vi "NHMFL TL Front Panel.vi"() -> ()   [LabVIEW 2020]
panel:
  out "Temp Display":enum32{"Helium 3", "VTI"}(tab)
  out "SORB":dbl
  out "1K POT":dbl
  out "3HE POT":dbl
  out "PROBE":dbl
  out "SAMPLE":dbl
  out "VTI":dbl
  in  "Load Probe Step Number":u8
  in  "Initialize":bool
  out "Array":dbl[][](array[numeric])
  in  "Menu Button":bool
  out "Tab Control":T1(tab)=enum."Menu"
  in  "Configure Instruments":bool
  in  "Choose Insert":enum32{"Helium 3", "VTI"}(radio)
  in  "Choose System":T2(radio)
  in  "Ring":u16(ring)=1 items=["Choose Function"=1, "He3 Condense"=3, "Change Setpoint"=8, "Temperature Ramp"=4]
  in  "stop":bool
  out "Load Probe Prompt":string
  in  "Load Probe: Next Step":bool
  out "Load Probe: Status":string
  in  "Quick Condense":bool
  in  "Condense Followup":u16(ring) items=["What Next?", "Hold @ 45K", "Run to Base", "Begin Ramp"]
  in  "Condense Continue Button":bool
  out "Position":string
  in  "Prior":bool
  in  "Next":bool
  in  "Soak Time":dbl format="%<%H:%M:%S>t"
  in  "Ramp Time":dbl format="%<%H:%M:%S>t"
  in  "Target Temp":dbl min=0.0 max=45.0 step=0.0001
  in  "Run Button":bool
  in  "Reset Button":bool
  out "Temp Array":dbl[](array[numeric])
  out "Time Array":dbl[][](array[numeric]) format="%<%H:%M:%S>t"
  in  "Proportional":sgl=1000.0 min=0 max=1000 step=0.1
  in  "Integral":sgl min=0 max=1000 step=0.1
  in  "Derivative":sgl min=0 max=1000 step=1
  out "Derivative Default":sgl
  out "Integral Default":sgl
  out "Proportional Default":sgl
  in  "Submit PID":bool
  in  "Probe Setpoint":dbl min=0.0 max=1.483 step=1e-05
  in  "Sorb Setpoint":dbl min=0.0 max=45.0 step=1e-05
  in  "Submit Setpoint":bool
  # "He3 Condensation:\n   Choose Full (1 hour) or Quick (30 min)\nCondense, then select a routine to start \nonce the helium has condensed."
  # "Condense,"
  # "then"
  # "Enter Target Sample Temperatures"
  # "Default"
  # "Change setpoint to what value?"
  # "≈"
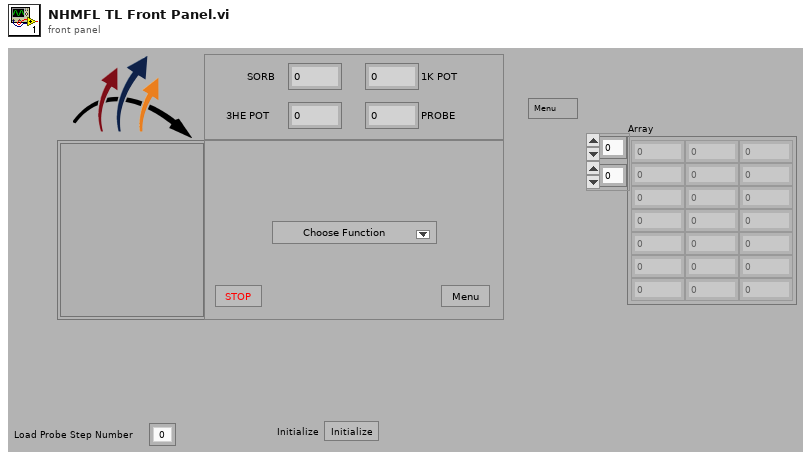
[diagram p1: front panel]
types:
  T1 = enum32{"Identify System", "Menu", "Load Probe", "He3 Condense", "Temperature Ramp", "Ramp Aray", "PID Control", "Configure Instruments", "Change Setpoint"}
  T2 = enum32{"TL-SC  (System A)", "SIV-32 (System B)", "TL-50  (System C)", "TL-32  (System D)"}
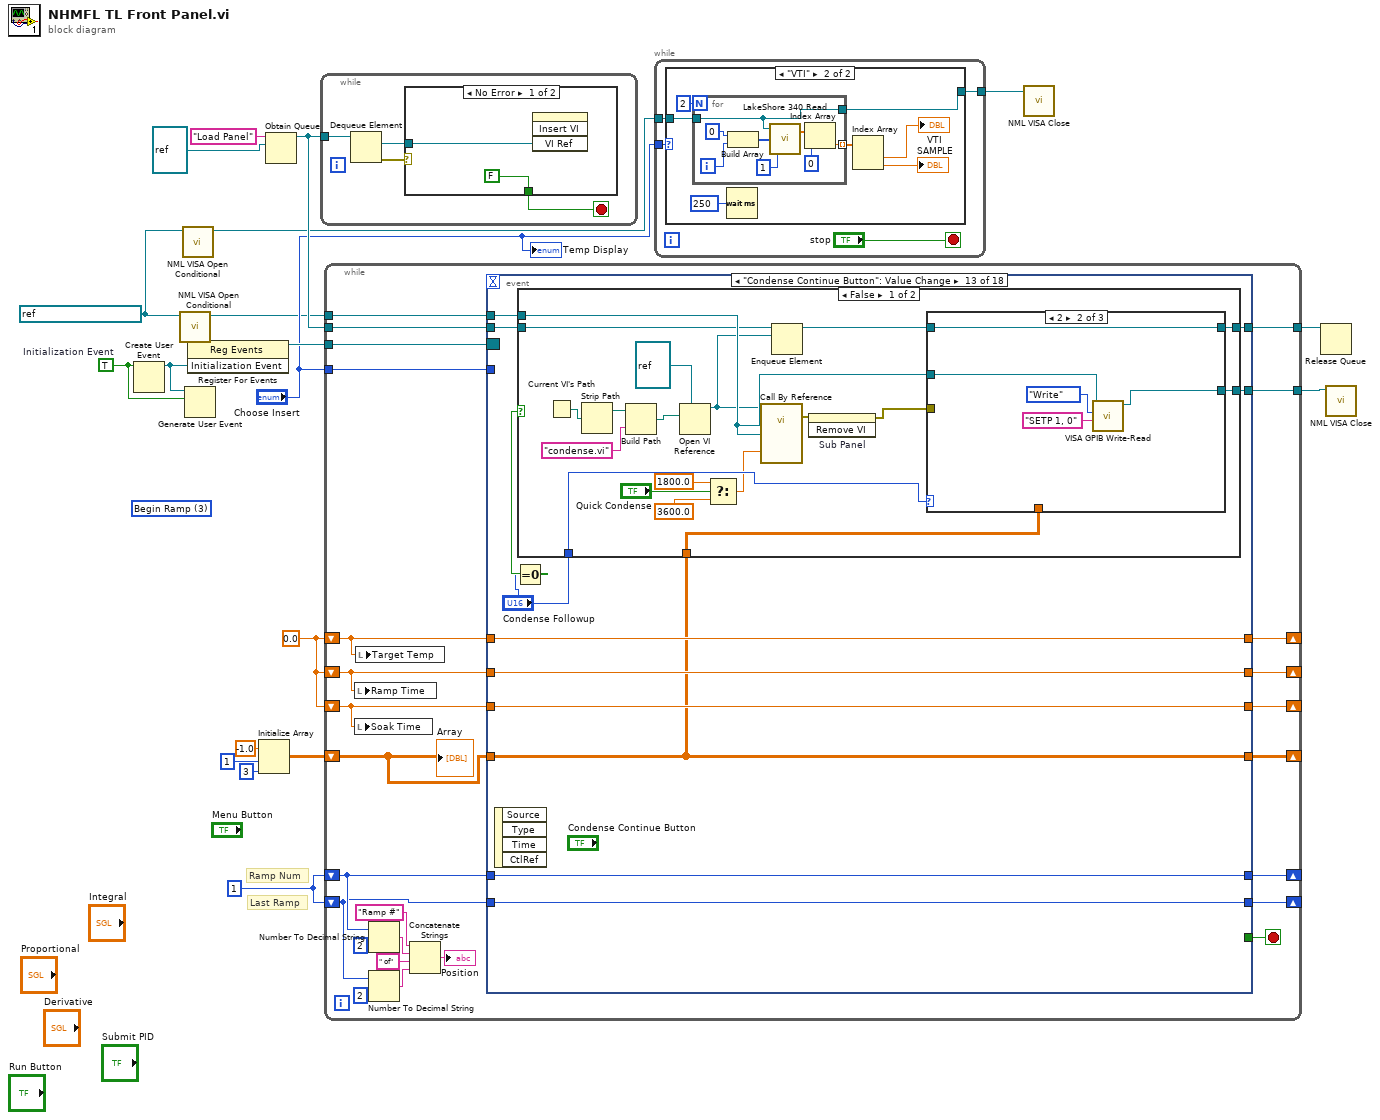
[diagram p0: block diagram]
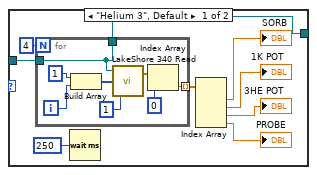
[diagram p2: hidden frame]
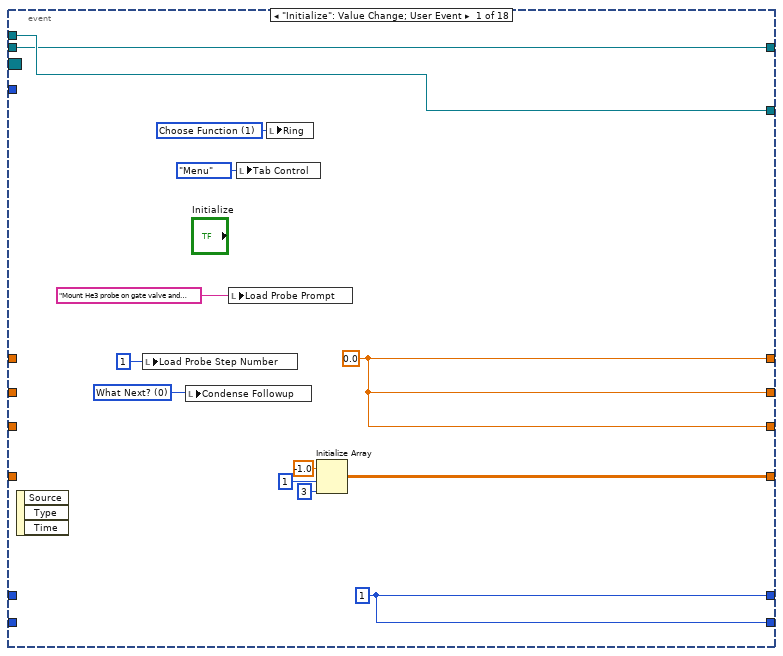
[diagram p3: hidden frame]
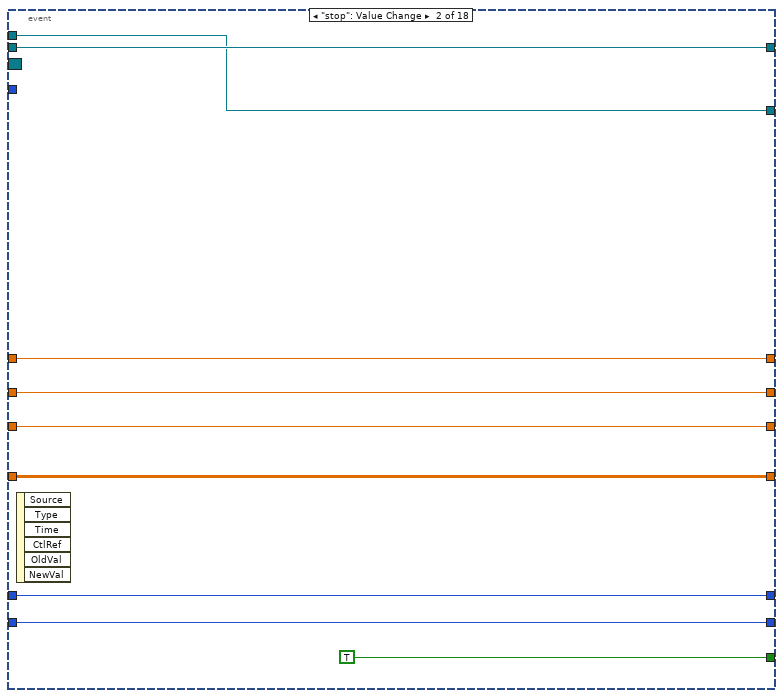
[diagram p4: hidden frame]
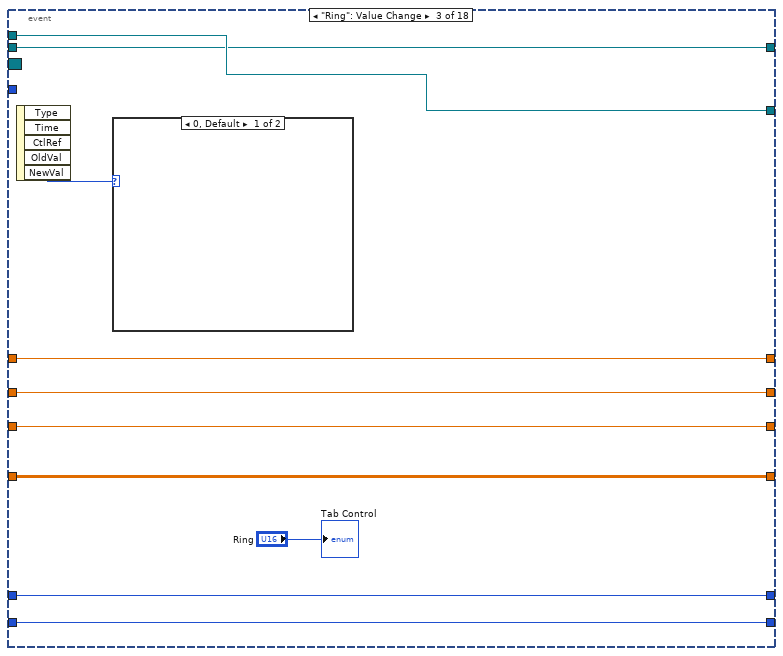
[diagram p5: hidden frame]
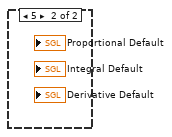
[diagram p6: hidden frame]
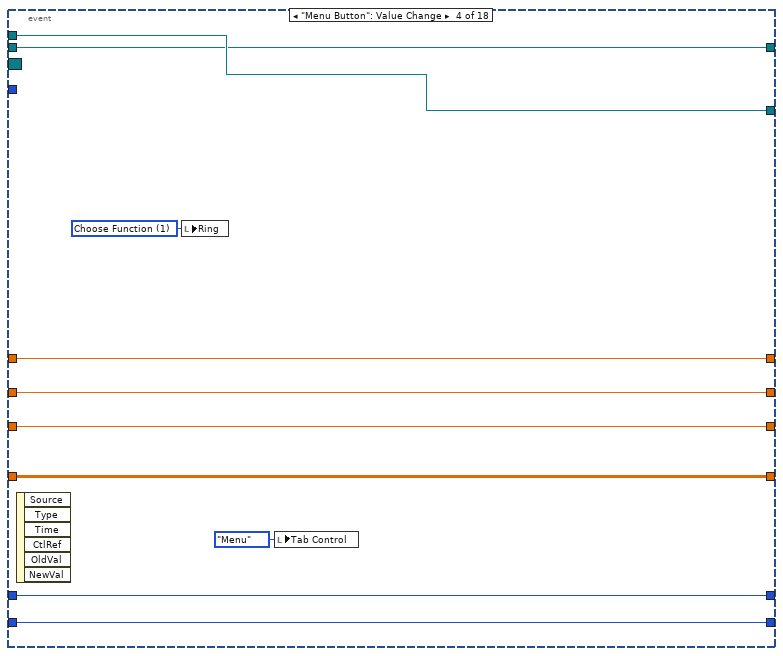
[diagram p7: hidden frame]
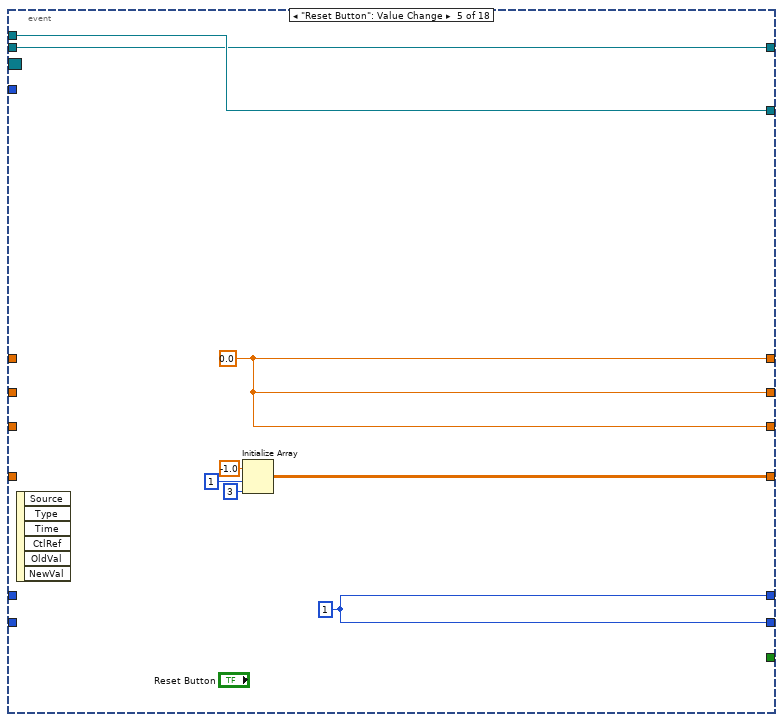
[diagram p8: hidden frame]
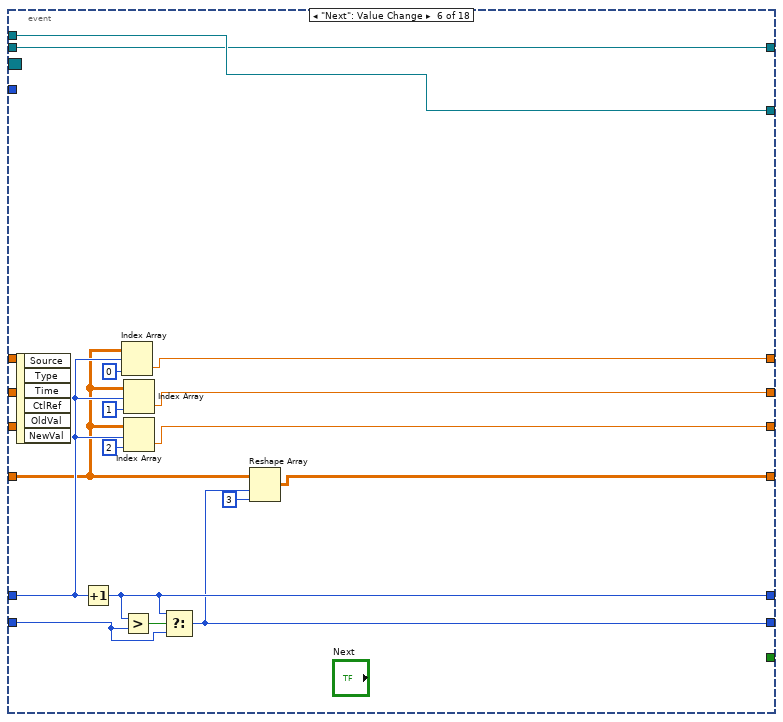
[diagram p9: hidden frame]
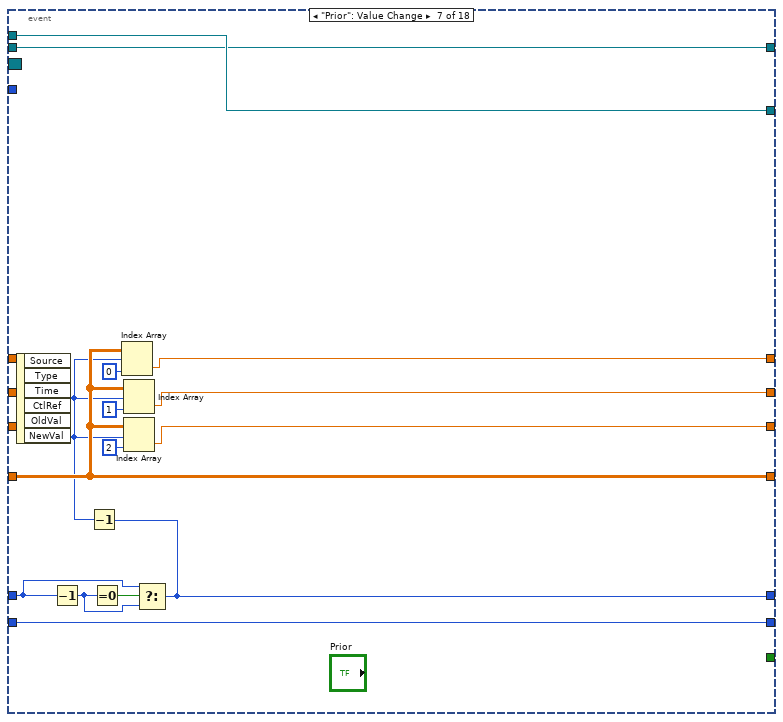
[diagram p10: hidden frame]
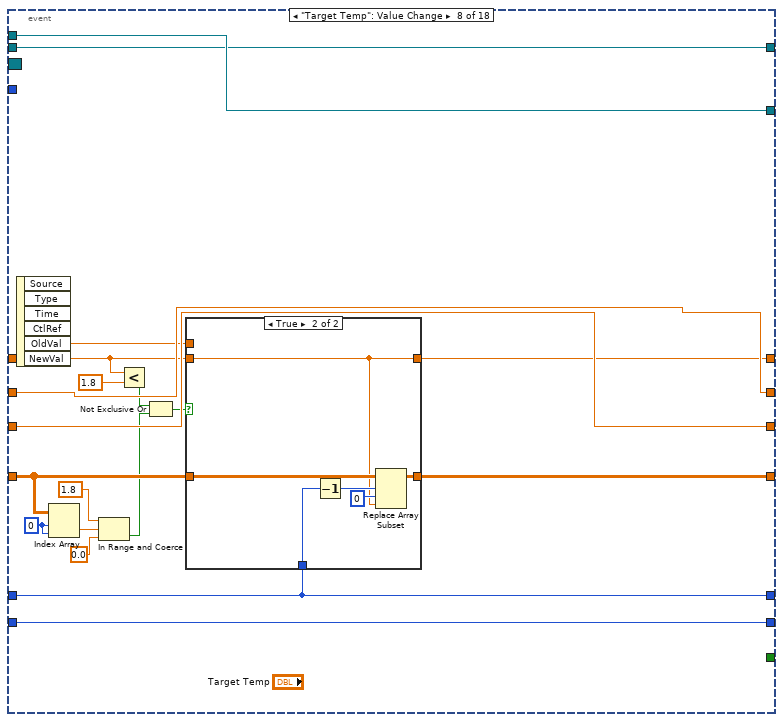
[diagram p11: hidden frame]
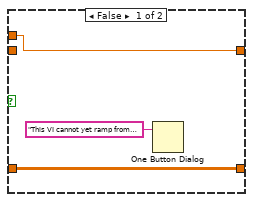
[diagram p12: hidden frame]
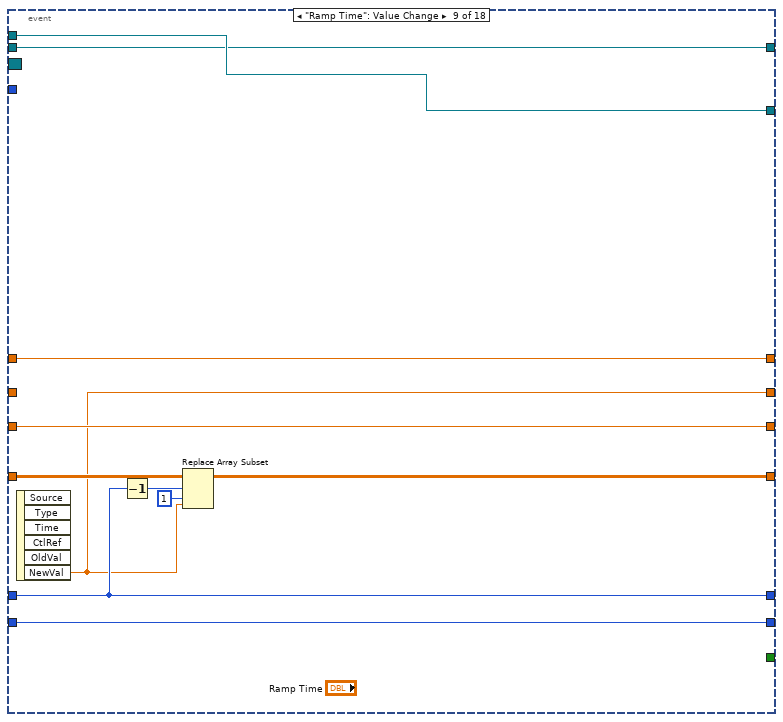
[diagram p13: hidden frame]
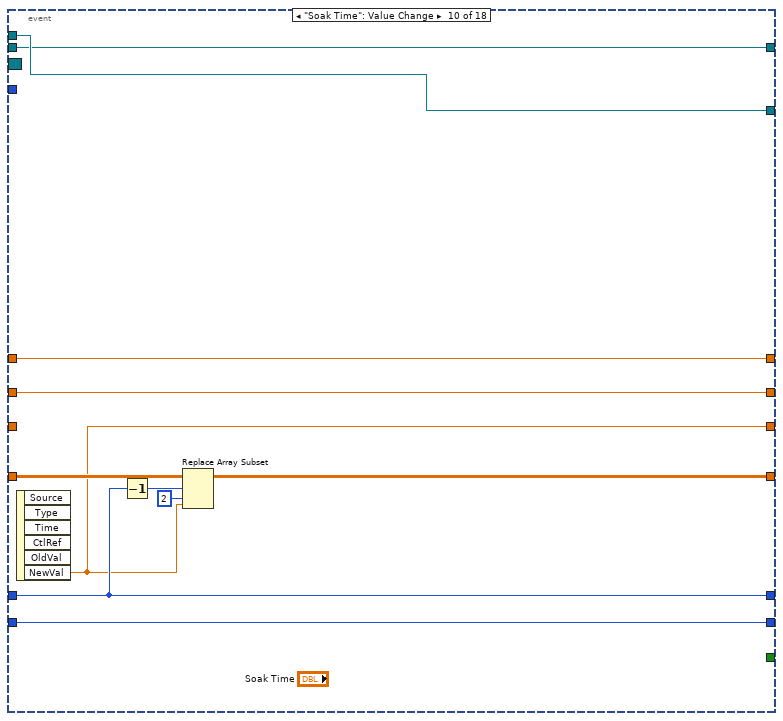
[diagram p14: hidden frame]
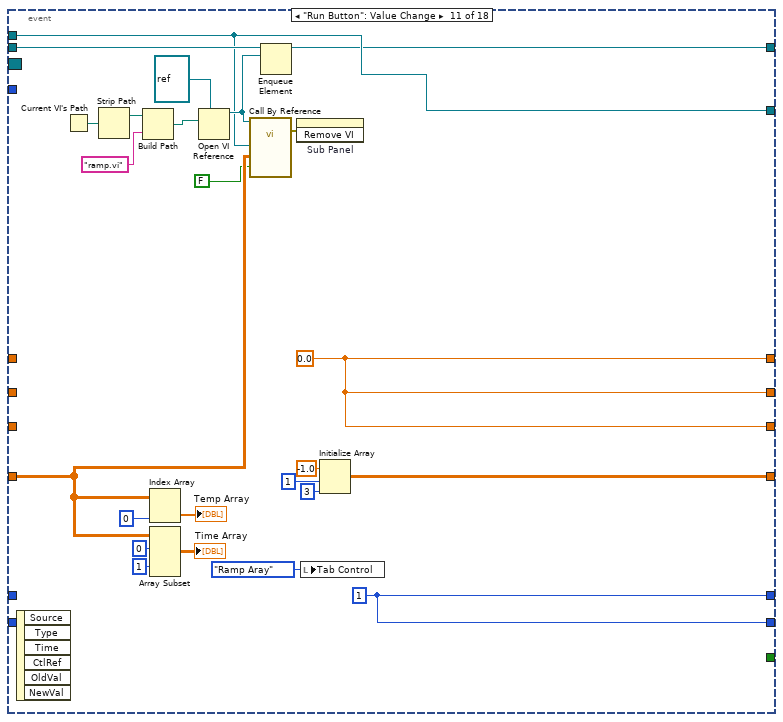
[diagram p15: hidden frame]
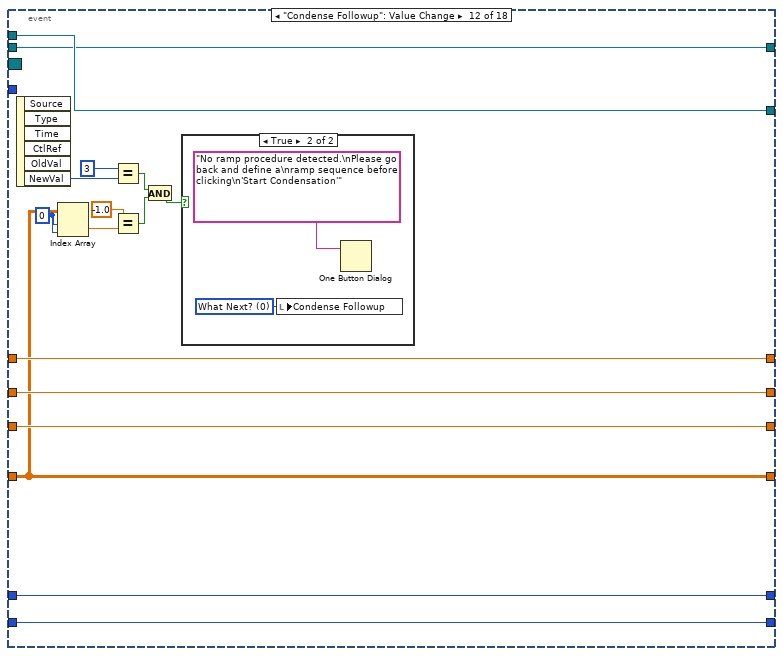
[diagram p16: hidden frame]
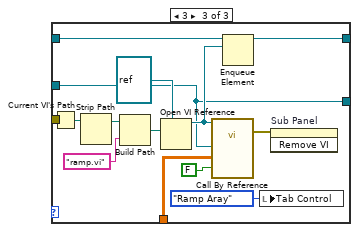
[diagram p19: hidden frame]
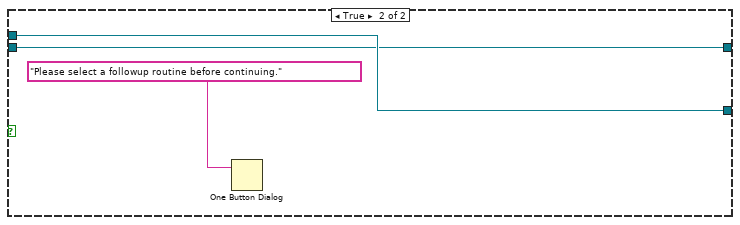
[diagram p20: hidden frame]
diagram:
  (unwired) u16 3 items=["What Next?", "Hold @ 40K", "Run to Base", "Begin Ramp"] ("Condense Followup")
  w7 = TRUE  # Initialization Event
  w6 = refnum<visa-resource-name> "GPIB0::12::INSTR" ("Instrument Address")
  w11 = u8 1
  w16 = 0.0 ("Target Temp")
  # "Last Ramp"
  # "Ramp Num"
  n1 = Create User Event(user event datatype=w7) -> (user event=w8:refnum<user-event>)  [unwired: 1 in, 1 out]
  n2 = call "NML VISA Open Conditional.vi"("VISA resource name"=w6) -> ("dup VISA Session"=w3:refnum<visa-resource-name>)  [unwired: 8 in, 2 out]
  n3 = call "NML VISA Open Conditional.vi"("VISA resource name"=w6) -> ("dup VISA Session"=w4:refnum<visa-resource-name>)  [unwired: 8 in, 2 out]
  n4 = Generate User Event(user event=w8, event data cluster=w7) -> ()  [unwired: 2 in, 2 out]
  n5 = register-events(w8) -> (reference out=w9:refnum<event-registration>)  [unwired: 2 in, 1 out]
  n6 = Initialize Array(-1.0 ("element"), 1 ("dimension size"), 3 ("dimension size")) -> (w12:dbl[][])
  n7 = Obtain Queue(name (unnamed)="Load Panel", element data type=refnum<vi> refnum ("vi reference")) -> (queue out=w17:refnum<queue>)  [unwired: 3 in, 2 out]
  n8 = while {
    tunnel: w17 -> [w23]
    stop <- w20 stop-if-true
    n9 = Dequeue Element(queue=w23) -> (element=w21:refnum<vi>, error out=w22:errorcluster)  [unwired: 2 in, 2 out]
    n10 = case shown="No Error" w22 {
      tunnel: w21 -> [w24 _]
      tunnel: [FALSE TRUE] -> w20
      frame No Error {
        n11 = invoke on="Sub Panel" class="SubPnl" method="Insert VI"("VI Ref"=w24) -> ()  [unwired: 3 in, 4 out]
      }
      frame Error {
      }
    }
  }
  n12 = while {
    tunnel: w17 -> [w33]
    shift-right: [w49] -> _
    shift-left: w12 -> [w31]
    shift-right: [w47] -> _
    shift-left: w16 -> [w50]
    shift-right: [w48] -> _
    shift-left: w16 -> [w51]
    shift-right: [w46] -> _
    shift-left: w16 -> [w52]
    shift-right: [w45] -> _
    shift-left: w11 -> [w36]
    shift-right: [w44] -> _
    shift-left: w11 -> [w35]
    tunnel: [w32] -> w10
    tunnel: w3 -> [w30]
    tunnel: w9 -> [w29]
    tunnel: "Choose Insert" -> [w28]
    tunnel: [w27] -> w1
    stop <- w34 stop-if-true
    n13 = local write "Ramp Time"(w51) -> ()
    n14 = local write "Soak Time"(w50) -> ()
    n15 = local write "Target Temp"(w52) -> ()
    n16 = Number To Decimal String(number=w36, width (-)=i16 2) -> (decimal integer string=w39:string)
    n17 = Number To Decimal String(number=w35, width (-)=i16 2) -> (decimal integer string=w37:string)
    n18 = Concatenate Strings("Ramp #", w39, " of", w37) -> (→"Position":string)
    n19 = event shown="[12] \"Condense Continue Button\": Value Change" {
      selector: w29 -> [_ _ _ _ _ _ _ _ _ _ _ _ _ _ _ _ _ _]
      dyn-events: _ -> [_ _ _ _ _ _ _ _ _ _ _ _ _ _ _ _ _ _]
      timeout: _ -> [_ _ _ _ _ _ _ _ _ _ _ _ _ _ _ _ _ _]
      tunnel: w51 -> [_ w70 w83 w93 _ _ _ w152 _ w176 _ w222 w233 w293 w325 w334 w344 w360]
      tunnel: w50 -> [_ w69 w82 w92 _ _ _ w151 w172 _ _ w221 w234 w292 w324 w333 w343 w359]
      tunnel: w52 -> [_ w71 w84 w94 _ _ _ _ w165 w177 _ w223 w232 w294 w326 w335 w345 w361]
      tunnel: w31 -> [_ w68 w81 w91 _ w105 w126 w147 w171 w183 w195 w216 w230 w291 w323 w332 w342 w358]
      tunnel: [w61 w68 w81 w91 w99 w109 w126 w150 w170 w182 w188 w216 w230 w291 w323 w332 w342 w358] -> w49
      tunnel: [w65 w70 w83 w93 w98 w107 w129 w152 w164 w176 w189 w222 w233 w293 w325 w334 w344 w360] -> w48
      tunnel: [w65 w69 w82 w92 w98 w115 w130 w151 w172 w175 w189 w221 w234 w292 w324 w333 w343 w359] -> w47
      tunnel: [w65 w71 w84 w94 w98 w106 w128 w140 w165 w177 w189 w223 w232 w294 w326 w335 w345 w361] -> w46
      tunnel: w35 -> [_ w66 w79 w89 _ w113 w127 w148 w166 w178 _ w219 w236 w289 w321 w330 w340 w356]
      tunnel: w36 -> [_ w67 w80 w90 _ w112 w124 w149 w167 w179 _ w220 w237 w290 w322 w331 w341 w357]
      tunnel: [w60 w67 w80 w90 w97 w111 w122 w149 w167 w179 w187 w220 w237 w290 w322 w331 w341 w357] -> w45
      tunnel: [w60 w66 w79 w89 w97 w108 w127 w148 w166 w178 w187 w219 w236 w289 w321 w330 w340 w356] -> w44
      tunnel: [_ TRUE _ _ _ _ _ _ _ _ _ _ _ _ _ _ _ _] -> w34
      tunnel: w33 -> [w53 w73 w75 w85 w95 w103 w119 w134 w162 w173 w196 w208 w235 w280 w312 w328 w338 w348]
      tunnel: [w53 w73 w75 w85 w95 w103 w119 w134 w162 w173 w184 w208 w226 w280 w312 w328 w338 w348] -> w32
      tunnel: w30 -> [w54 w72 w76 w86 w96 w104 w120 w135 w163 w174 w185 w209 w231 w281 w313 w329 w339 w351]
      tunnel: w28 -> [_ _ _ _ _ _ _ _ _ _ _ _ _ _ w318 _ _ _]
      tunnel: [w54 w72 w76 w86 w96 w104 w120 w135 w163 w174 w185 w209 w227 w281 w313 w329 w339 w350] -> w27
      event "Initialize": Value Change; User Event {
        w55 = u16 1 items=["Choose Function"=1, "He3 Condense"=3, "Change Setpoint"=8, "Temperature Ramp"=4] ("Ring")
        w57 = u16 0 items=["What Next?", "Hold @ 45K", "Run to Base", "Begin Ramp"] ("Condense followup")
        w60 = u8 1
        w65 = 0.0 ("Target Temp")
        n20 = event-data() -> ()  [unwired: 1 in, 3 out]
        n21 = local write "Load Probe Step Number"(u8 1 ("Load Probe Step Number")) -> ()
        n22 = local write "Condense Followup"(w57) -> ()
        n23 = local write "Load Probe Prompt"("Mount He3 probe on gate valve and tighten KF-50 clamp." ("Load Probe Prompt")) -> ()
        n24 = local write "Tab Control"(T1."Menu" ("Tab Control")) -> ()
        n25 = local write "Ring"(w55) -> ()
        n26 = Initialize Array(-1.0 ("element"), 1 ("dimension size"), 3 ("dimension size")) -> (w61:dbl[][])
      }
      event "stop": Value Change {
        n27 = event-data() -> ()  [unwired: 1 in, 6 out]
      }
      event "Ring": Value Change {
        n28 = event-data() -> ("NewVal"=w77:u16)  [unwired: 1 in, 4 out]
        n29 = case shown="0, Default" w77 {
          frame 0, Default {
          }
          frame 5 {
          }
        }
        "Tab Control" <- "Ring"
      }
      event "Menu Button": Value Change {
        w87 = u16 1 items=["Choose Function"=1, "He3 Condense"=3, "Change Setpoint"=8, "Temperature Ramp"=4] ("Ring")
        n30 = event-data() -> ()  [unwired: 1 in, 6 out]
        n31 = local write "Ring"(w87) -> ()
        n32 = local write "Tab Control"(T1."Menu" ("Tab Control")) -> ()
      }
      event "Reset Button": Value Change {
        w97 = u8 1
        w98 = 0.0 ("Target Temp")
        n33 = event-data() -> ()  [unwired: 1 in, 6 out]
        n34 = Initialize Array(-1.0 ("element"), 1 ("dimension size"), 3 ("dimension size")) -> (w99:dbl[][])
      }
      event "Next": Value Change {
        n35 = event-data() -> ()  [unwired: 1 in, 6 out]
        n36 = Increment(x=w112) -> (x+1=w111:u8)
        n37 = Index Array(array=w105, index (row)=w112, index (col)=0 ("disabled index (col)")) -> (element=w106:dbl)
        n38 = Greater?(x=w111, y=w113) -> (0:w114:bool)
        n39 = Index Array(array=w105, index (row)=w112, index (col)=1 ("disabled index (col)")) -> (element=w107:dbl)
        n40 = Index Array(array=w105, index (row)=w112, index (col)=2 ("disabled index (col)")) -> (element=w115:dbl)
        n41 = Select(t=w111, s=w114, f=w113) -> (s? t:f=w108:u8)
        n42 = Reshape Array(w105, w108, 3 ("dimension size")) -> (w109:dbl[][])
      }
      event "Prior": Value Change {
        n43 = event-data() -> ()  [unwired: 1 in, 6 out]
        n44 = Decrement(x=w124) -> (x-1=w123:u8)
        n45 = Equal To 0?(x=w123) -> (x = 0?=w125:bool)
        n46 = Select(t=w124, s=w125, f=w123) -> (s? t:f=w122:u8)
        n47 = Decrement(x=w122) -> (x-1=w121:u8)
        n48 = Index Array(array=w126, index (row)=w121, index (col)=0 ("disabled index (col)")) -> (element=w128:dbl)
        n49 = Index Array(array=w126, index (row)=w121, index (col)=1 ("disabled index (col)")) -> (element=w129:dbl)
        n50 = Index Array(array=w126, index (row)=w121, index (col)=2 ("disabled index (col)")) -> (element=w130:dbl)
      }
      event "Target Temp": Value Change {
        w146 = 0 ("index (row)")
        n51 = event-data() -> ("OldVal"=w141:dbl, "NewVal"=w143:dbl)  [unwired: 1 in, 4 out]
        n52 = Index Array(array=w147, index (row)=w146, index (col)=w146) -> (element=w139:dbl)
        n53 = In Range and Coerce(upper limit=1.8 ("y"), x=w139, lower limit=0.0) -> (In Range?=w136:bool)  [unwired: 1 out]
        n54 = Less?(x=w143, y=1.8) -> (x < y?=w144:bool)
        n55 = Not Exclusive Or(1:w136, 2:w144) -> (0:w142:bool)
        n56 = case shown="True" w142 {
          tunnel: [w154 w161] -> w150
          tunnel: w149 -> [_ w160]
          tunnel: w147 -> [w154 w159]
          tunnel: w143 -> [_ w156]
          tunnel: w141 -> [w155 _]
          tunnel: [w155 w156] -> w140
          frame False {
            n57 = One Button Dialog(message="This VI cannot yet ramp from low-temperature (Probe < 1.8K) to high temperature modes.\n\nPlease use two seperate ramp routines.") -> ()  [unwired: 1 in, 1 out]
          }
          frame True {
            n58 = Decrement(x=w160) -> (x-1=w157:u8)
            n59 = Replace Array Subset(array=w159, new element=w156, index (row)=w157, index (col)=0 ("disabled index (col)")) -> (w161:dbl[][])
          }
        }
      }
      event "Ramp Time": Value Change {
        n60 = event-data() -> ("NewVal"=w164:dbl)  [unwired: 1 in, 5 out]
        n61 = Decrement(x=w167) -> (x-1=w168:u8)
        n62 = Replace Array Subset(array=w171, new element=w164, index (row)=w168, index (col)=1 ("disabled index (col)")) -> (w170:dbl[][])
      }
      event "Soak Time": Value Change {
        n63 = event-data() -> ("NewVal"=w175:dbl)  [unwired: 1 in, 5 out]
        n64 = Decrement(x=w179) -> (x-1=w180:u8)
        n65 = Replace Array Subset(array=w183, new element=w175, index (row)=w180, index (col)=2 ("disabled index (col)")) -> (w182:dbl[][])
      }
      event "Run Button": Value Change {
        w187 = u8 1
        w189 = 0.0 ("Target Temp")
        n66 = event-data() -> ()  [unwired: 1 in, 6 out]
        n67 = Current VI's Path() -> (path=w197:path)
        n68 = Strip Path(path=w197) -> (stripped path=w201:path)  [unwired: 1 out]
        n69 = Build Path(base path=w201, name or relative path="ramp.vi") -> (appended path=w200:path)
        n70 = Index Array(array=w195, index (col)=0 ("index (row)")) -> (element=→"Temp Array":dbl[])  [unwired: 1 in]
        n71 = Array Subset(array=w195, index (row)=0, index (col)=1 ("index")) -> (→"Time Array":dbl[][])  [unwired: 2 in]
        n72 = Open VI Reference(type specifier VI Refnum (for type only)=refnum<vi> refnum, vi path=w200) -> (vi reference=w199:refnum<vi>)  [unwired: 4 in, 1 out]
        n73 = call-by-ref "?"(reference=w199, "Log Scale?"=FALSE, "Array"=w195, "Instrument Address"=w185) -> (error out=w194:errorcluster)  [unwired: 1 in, 1 out]
        n74 = Enqueue Element(queue=w196, element=w199) -> (queue out=w184:refnum<queue>)  [unwired: 2 in, 2 out]
        n75 = invoke on="Sub Panel" class="SubPnl" method="Remove VI"(error in=w194) -> ()  [unwired: 2 in, 3 out]
        n76 = local write "Tab Control"(T1."Ramp Aray" ("Tab Control")) -> ()
        n77 = Initialize Array(-1.0 ("element"), 1 ("dimension size"), 3 ("dimension size")) -> (w188:dbl[][])
      }
      event "Condense Followup": Value Change {
        w215 = 0 ("index (row)")
        n78 = event-data() -> ("NewVal"=w218:u16)  [unwired: 1 in, 5 out]
        n79 = Index Array(array=w216, index (row)=w215, index (col)=w215) -> (element=w214:dbl)
        n80 = Equal?(x=u16 3, y=w218) -> (x = y?=w211:bool)
        n81 = Equal?(x=-1.0, y=w214) -> (x = y?=w212:bool)
        n82 = And(x=w211, y=w212) -> (x .and. y?=w210:bool)
        n83 = case shown="True" w210 {
          frame False {
          }
          frame True {
            w224 = u16 0 items=["What Next?", "Hold @ 40K", "Run to Base", "Begin Ramp"] ("Condense Followup")
            n84 = local write "Condense Followup"(w224) -> ()
            n85 = One Button Dialog(message="No ramp procedure detected.\nPlease go back and define a\nramp sequence before clicking\n'Start Condensation'") -> ()  [unwired: 1 in, 1 out]
          }
        }
      }
      event "Condense Continue Button": Value Change {
        n86 = event-data() -> ()  [unwired: 1 in, 4 out]
        n87 = Equal To 0?(x="Condense Followup") -> (x = 0?=w229:bool)
        n88 = case shown="False" w229 {
          tunnel: w235 -> [w240 w277]
          tunnel: w231 -> [w256 w278]
          tunnel: w230 -> [w255 _]
          tunnel: "Condense Followup" -> [w254 _]
          tunnel: [w253 w278] -> w227
          tunnel: [w238 w277] -> w226
          frame False {
            n89 = Current VI's Path() -> (path=w252:path)
            n90 = Strip Path(path=w252) -> (stripped path=w244:path)  [unwired: 1 out]
            n91 = Build Path(base path=w244, name or relative path="condense.vi") -> (appended path=w245:path)
            n92 = Open VI Reference(type specifier VI Refnum (for type only)=refnum<vi> refnum, vi path=w245) -> (vi reference=w250:refnum<vi>)  [unwired: 4 in, 1 out]
            n93 = Select(t=1800.0, s="Quick Condense", f=3600.0 ("t")) -> (s? t:f=w242:dbl)
            n94 = call-by-ref "?"(reference=w250, "Time"=w242, "GPIB Address"=w256) -> (error out=w246:errorcluster)  [unwired: 2 in, 1 out]
            n95 = Enqueue Element(queue=w240, element=w250) -> (queue out=w239:refnum<queue>)  [unwired: 2 in, 2 out]
            n96 = invoke on="Sub Panel" class="SubPnl" method="Remove VI"(error in=w246) -> (error out=w241:errorcluster)  [unwired: 2 in, 2 out]
            n97 = case shown="2" w254 {
              tunnel: w256 -> [w258 w262 w265]
              tunnel: w239 -> [w257 w260 w268]
              tunnel: w255 -> [_ _ w267]
              tunnel: [w258 w261 w265] -> w253
              tunnel: w241 -> [_ _ _]
              tunnel: [w257 w260 w264] -> w238
              frame 0, Default {
              }
              frame 2 {
                n98 = call "VISA GPIB Write-Read.vi"("Command"="SETP 1, 0" ("Command String"), "Action"=enum16{"Write", "Read", "Write & Read"}."Write", "VISA resource name"=w262) -> ("dup VISA Session"=w261:refnum<visa-resource-name>)  [unwired: 5 in, 3 out]
              }
              frame 3 {
                n99 = Current VI's Path() -> (path=w274:path)
                n100 = Strip Path(path=w274) -> (stripped path=w270:path)  [unwired: 1 out]
                n101 = Build Path(base path=w270, name or relative path="ramp.vi") -> (appended path=w271:path)
                n102 = Open VI Reference(type specifier VI Refnum (for type only)=refnum<vi> refnum, vi path=w271) -> (vi reference=w272:refnum<vi>)  [unwired: 4 in, 1 out]
                n103 = call-by-ref "?"(reference=w272, "Log Scale?"=FALSE, "Array"=w267, "Instrument Address"=w265) -> (error out=w275:errorcluster)  [unwired: 1 in, 1 out]
                n104 = Enqueue Element(queue=w268, element=w272) -> (queue out=w264:refnum<queue>)  [unwired: 2 in, 2 out]
                n105 = local write "Tab Control"(T1."Ramp Aray" ("Tab Control")) -> ()
                n106 = invoke on="Sub Panel" class="SubPnl" method="Remove VI"(error in=w275) -> ()  [unwired: 2 in, 3 out]
              }
            }
          }
          frame True {
            n107 = One Button Dialog(message="Please select a followup routine before continuing.") -> ()  [unwired: 1 in, 1 out]
          }
        }
      }
      event "Load Probe: Next Step": Value Change {
        n108 = event-data() -> ()  [unwired: 1 in, 6 out]
        n109 = case shown="17" "Load Probe Step Number" {
          tunnel: [_ _ _ "Mount 3He probe on gate valve and tighten KF-50 clamp." "Connect Turbo Pump pumping line to the probe load lock and tighten KF-16 clamp." "Open Load Lock Valve." "Open Sliding Seal Valve." "Open Pump Valve." "Turn on Turbo Pump and pump out the load lock until the pressure reaches 5e-3 mbar." "Connect probe sensor cables to probe connector and Lakeshore 340 Temperature Controller, input channel \"D\"." "After the pressure reaches 5e-3 mbar, close Lode Lock Valve." "Open Gate Valve." "Hold probe and loosen probe clamp." "Lower probe until the bottom of the probe head is about 36 inches from the top of the load lock and tighten probe clamp." "Set Sorb temperature ti 25K and heater output to 25W on Lakeshore 340 Temperature Controller." "Observe the Lakeshore 340 Temperature Controller digital display.  When output channel \"D\" reache approximately 4K or 1.1 Kohm" "Hold probe and loosen probe clamp and lower the probe.  When lowering the probe observe the temperature on output channel \"D\", it should start to increase.  Keep lowering the probe until the temperature starts to decrease, stop and tighten probe clamp." "Wait 10 minutes for 4K Heat Sink to cool." "Hold probe and remove probe clamp.  Insert the probe all the way." "Hand-tighten 4K Heat Sink Lock Down Nut on top of probe load lock and back off 1/4 turn.  Probe shaft will differentially expand relative to cryostat and probe will 'lock' in place.  Hense backing off 1/4 turn of the 4K"] -> w282
          frame 0, Default {
          }
          frame 1 {
          }
          frame 2 {
          }
          frame 3 {
          }
          frame 4 {
          }
          frame 5 {
          }
          frame 6 {
          }
          frame 7 {
          }
          frame 8 {
          }
          frame 9 {
          }
          frame 10 {
          }
          frame 11 {
          }
          frame 12 {
          }
          frame 13 {
          }
          frame 14 {
          }
          frame 15 {
          }
          frame 16 {
          }
          frame 17 {
          }
          frame 18 {
          }
          frame 19 {
          }
        }
        "Load Probe Prompt" <- w282
        n110 = Number To Decimal String(number="Load Probe Step Number", width (-)=i16 2) -> (decimal integer string=w287:string)
        n111 = Concatenate Strings("Step #", w287, " of X") -> (→"Load Probe: Status":string)
      }
      event "Configure Instruments": Value Change {
        n112 = event-data() -> ()  [unwired: 1 in, 6 out]
        n113 = Equal?(x=enum32{"Helium 3", "VTI"}."Helium 3" ("Choose Insert"), y=w318) -> (x = y?=w316:bool)
        n114 = Equal?(x=T2."SIV-32 (System B)" ("Choose System"), y="Choose System") -> (x = y?=w315:bool)
        n115 = And(x=w316, y=w315) -> (x .and. y?=w314:bool)
        n116 = case shown="False" w314 {
          frame False {
            n117 = One Button Dialog(message="This VI currently only supports System B with He3 insert.") -> ()  [unwired: 1 in, 1 out]
          }
          frame True {
          }
        }
      }
      event "Sorb Setpoint": Value Change {
        n118 = event-data() -> ("NewVal"=w337:dbl)  [unwired: 1 in, 5 out]
        n119 = call "System A Temp Curve.vi"("Sorb Goal Temp"=w337) -> ("Corresponding He3 Temp"=w336:dbl)  [unwired: 1 in, 1 out]
        n120 = local write "Probe Setpoint"(w336) -> ()
      }
      event "Probe Setpoint": Value Change {
        n121 = event-data() -> ("NewVal"=w347:dbl)  [unwired: 1 in, 5 out]
        n122 = call "System A Temp Curve.vi"("He3 Goal Temp"=w347) -> ("Corresponding Sorb Temp"=w346:dbl)  [unwired: 1 in, 1 out]
        n123 = local write "Sorb Setpoint"(w346) -> ()
      }
      event "Submit Setpoint": Value Change {
        n124 = event-data() -> ()  [unwired: 1 in, 6 out]
        n125 = Number To Fractional String(number="Sorb Setpoint") -> (F-format string=w355:string)  [unwired: 3 in]
        n126 = Concatenate Strings("SETP 1, " ("String to Write"), w355) -> (w353:string)
        n127 = call "VISA GPIB Write-Read.vi"("Command"=w353, "Action"=enum16{"Write", "Read", "Write & Read"}."Write", "VISA resource name"=w351) -> ("dup VISA Session"=w350:refnum<visa-resource-name>)  [unwired: 5 in, 3 out]
      }
    }
    "Array" <- w31
  }
  n128 = while {
    tunnel: w4 -> [w365]
    tunnel: "Choose Insert" -> [w364]
    tunnel: [w362] -> w2
    stop <- "stop" stop-if-true
    n129 = case shown="\"VTI\"" w364 {
      tunnel: w365 -> [w374 w389]
      tunnel: [w366 w383] -> w362
      frame "Helium 3", Default {
        n130 = for {
          N: 4 -> [_]
          tunnel: w374 -> [w375]
          tunnel: [w376] -> w371 mode=indexing
          tunnel: [w375] -> w366
          i -> [w378]
          n131 = Build Array(1, w378) -> (w377:i32[])
          n132 = call "LakeShore 340 Read.vi"("Point #"=1, "Parameters"=w377, "Instrument Address"=w375) -> ("Measurement"=w381:dbl[])  [unwired: 1 out]
          n133 = Index Array(array=w381, index=0) -> (element=w376:dbl)
        }
        n134 = Wait (ms)(milliseconds to wait=u32 250) -> ()  [unwired: 1 out]
        n135 = Index Array(array=w371) -> (element #1=→"SORB":dbl, element #2=→"1K POT":dbl, element #3=→"3HE POT":dbl, element #4=→"PROBE":dbl)  [unwired: 4 in]
      }
      frame "VTI" {
        n136 = for {
          N: 2 -> [_]
          tunnel: w389 -> [w390]
          tunnel: [w391] -> w386 mode=indexing
          tunnel: [w390] -> w383
          i -> [w393]
          n137 = Build Array(0, w393) -> (w392:i32[])
          n138 = call "LakeShore 340 Read.vi"("Point #"=1, "Parameters"=w392, "Instrument Address"=w390) -> ("Measurement"=w396:dbl[])  [unwired: 1 out]
          n139 = Index Array(array=w396, index=0) -> (element=w391:dbl)
        }
        n140 = Wait (ms)(milliseconds to wait=u32 250) -> ()  [unwired: 1 out]
        n141 = Index Array(array=w386) -> (element #1=→"VTI":dbl, element #2=→"SAMPLE":dbl)  [unwired: 2 in]
      }
    }
  }
  n142 = call "NML VISA Close.vi"("VISA resource name"=w2) -> ()  [unwired: 10 in, 1 out]
  n143 = Release Queue(queue=w10) -> ()  [unwired: 2 in, 3 out]
  n144 = call "NML VISA Close.vi"("VISA resource name"=w1) -> ()  [unwired: 10 in, 1 out]
  "Temp Display" <- "Choose Insert"
